vi "sendTel.vi"(8 "error in (no error)":errorcluster, 9 "queueOptions":T1={"EnqueueOptions"=enum."normal enqueue", "Timeout"=0}, 10 "Telemetry":T3, 11 "tcpServer in":refnum<class "TcpServer.lvclass">) -> (0 "error out":errorcluster, 3 "tcpServer out":refnum<class "TcpServer.lvclass">)   [LabVIEW 2018, in "TcpServer.lvclass"]
doc: "Send telemetry to TCP Client. Use the queueOptions control to select lossy enqueue or normal enqueue, and timeout in ms."
uses:
  TcpServer.lvclass
  TcpServerTel/typedef/telTypeDef.ctl
  TcpServerTel/typedef/queueOptionsTypeDef.ctl
  TcpServerTel/typedef/enqueueOptionsTypeDef.ctl
  TcpServer.lvclass/TcpServer.ctl
  TcpServerTel/TcpServerTel.lvclass
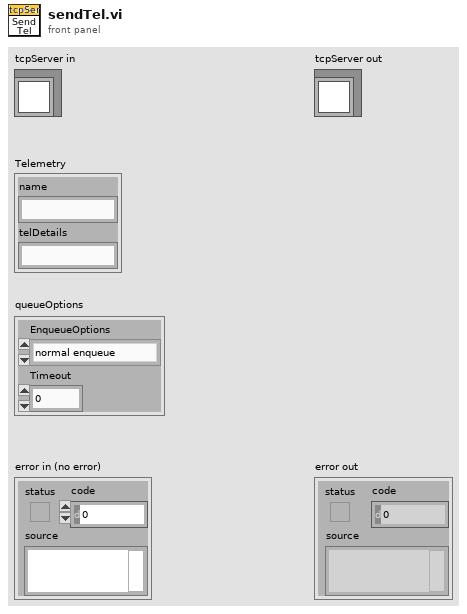
[diagram p1: front panel]
types:
  T1 = typedef "TcpServerTel.lvclass/queueOptionsTypeDef.ctl" = cluster{"EnqueueOptions":T2, "Timeout":i32}
  T2 = typedef "TcpServerTel.lvclass/enqueueOptionsTypeDef.ctl" = enum16{"lossy enqueue", "normal enqueue"}
  T3 = typedef "TcpServerTel.lvclass/telTypeDef.ctl" = cluster{"name":string, "telDetails":string}
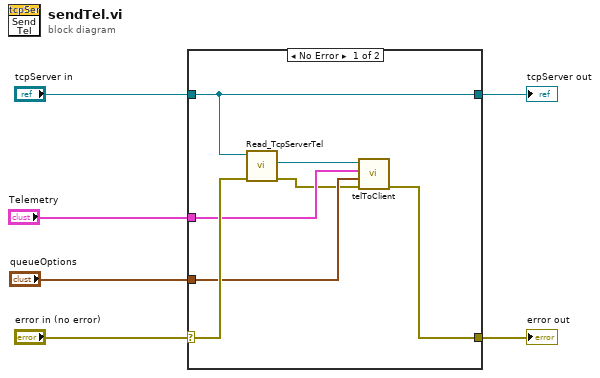
[diagram p0: block diagram]
diagram:
  n1 = case shown="No Error" "error in (no error)" {
    selector: "error in (no error)" -> [w13 w15]
    tunnel: [w7 w15] -> w5
    tunnel: "tcpServer in" -> [w12 w14]
    tunnel: [w12 w14] -> w3
    tunnel: "Telemetry" -> [w10 _]
    tunnel: "queueOptions" -> [w9 _]
    frame No Error {
      n2 = call "Read_TcpServerTel.vi"("error in (no error)"=w13, "TcpServer in"=w12) -> ("error out"=w8:errorcluster, "TcpServerTel.lvclass"=w11:refnum<class "TcpServerTel.lvclass">)  [unwired: 7 in, 1 out]
      n3 = call "telToClient.vi"("error in (no error)"=w8, "queueOptions"=w9, "Telemetry"=w10, "TcpServerTel in"=w11) -> ("error out"=w7:errorcluster)  [unwired: 6 in, 1 out]
    }
    frame Error {
    }
  }
  "error out" <- w5
  "tcpServer out" <- w3
